vi "extended.vi"(1 "Numeric Input":ext format="%.2f") -> (0 "Numeric Output":ext format="%.2f")   [LabVIEW 2010]
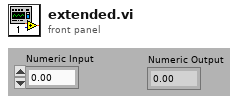
[diagram p1: front panel]
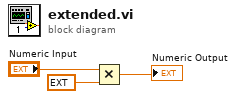
[diagram p0: block diagram]
diagram:
  n1 = Multiply(x="Numeric Input", y=ext 2.0) -> (x*y=→"Numeric Output":ext)
